vi "getSampleRate.vi"(1 "Number of active channels":i32) -> (0 "Sample Rate":dbl=1000000.0)   [LabVIEW 2013]
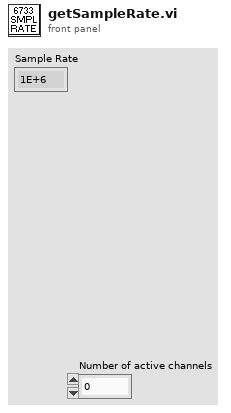
[diagram p1: front panel]
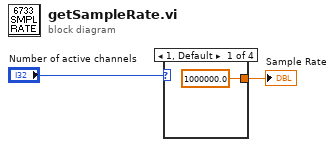
[diagram p0: block diagram]
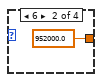
[diagram p2: hidden frame]
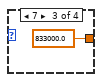
[diagram p3: hidden frame]
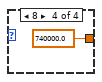
[diagram p4: hidden frame]
diagram:
  n1 = case shown="1, Default" "Number of active channels" {
    tunnel: [1000000.0 952000.0 833000.0 740000.0] -> w1
    frame 1, Default {
    }
    frame 6 {
    }
    frame 7 {
    }
    frame 8 {
    }
  }
  "Sample Rate" <- w1
